vi "Init.vi"(8 "error in (no error)":errorcluster, 10 "model_v1_parameters":T1, 11 "OUR_Monitor in":refnum<class "OUR_Monitor.lvclass">) -> (0 "error out":errorcluster, 3 "OUR_Monitor out":refnum<class "OUR_Monitor.lvclass">)   [LabVIEW 2021, in "MBPOnOff_Controller.lvlib" / "OUR_Monitor.lvclass"]
uses:
  OUR_Monitor.lvclass
  Model_Predictor/typedefs/Model_v1_parameters.ctl
  OUR_Monitor.lvclass/OUR_Monitor.ctl
  Model_Predictor/Model_Predictor.lvclass
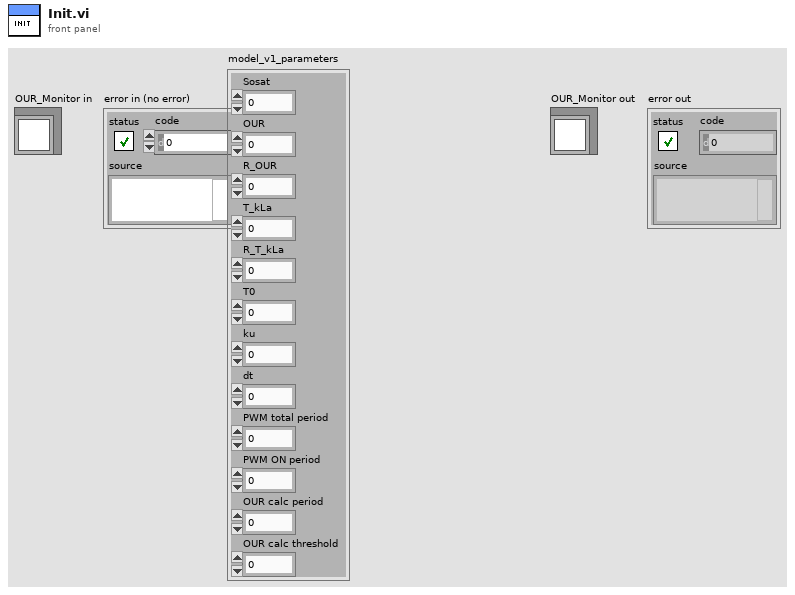
[diagram p1: front panel]
types:
  T1 = typedef "MBPOnOff_Controller.lvlib/Model_Predictor.lvclass/Model_v1_parameters.ctl" = cluster{"Sosat":dbl, "OUR":dbl, "R_OUR":dbl, "T_kLa":dbl, "R_T_kLa":dbl, "T0":dbl, "ku":dbl, "dt":dbl, "PWM total period":dbl, "PWM ON period":dbl, "OUR calc period":dbl, "OUR calc threshold":dbl}
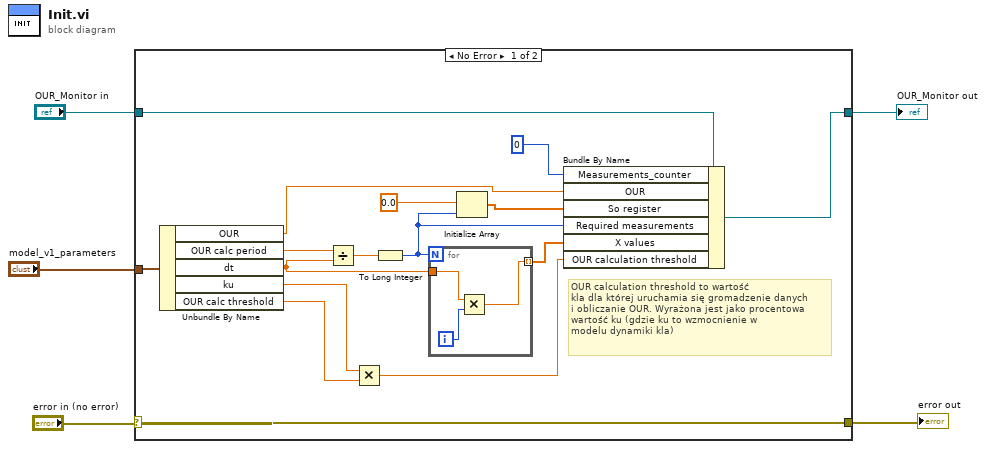
[diagram p0: block diagram]
diagram:
  n1 = case shown="No Error" "error in (no error)" {
    selector: "error in (no error)" -> [w21 w26]
    tunnel: [w21 w26] -> w4
    tunnel: [w17 w25] -> w3
    tunnel: "OUR_Monitor in" -> [w20 w25]
    tunnel: "model_v1_parameters" -> [w11 _]
    frame No Error {
      # "OUR calculation threshold to wartość\nkla dla której uruchamia się gromadzenie danych\ni obliczanie OUR. Wyrażona jest jako procentowa \nwartość ku (gdzie ku to wzmocnienie w\nmodelu dynamiki kla)"
      n2 = Unbundle By Name(w11) -> ("OUR"=w10:dbl, "OUR calc period"=w9:dbl, "dt"=w6:dbl, "ku"=w8:dbl, "OUR calc threshold"=w7:dbl)
      n3 = Divide(x=w9, y=w6) -> (x/y=w18:dbl)
      n4 = Multiply(x=w8, y=w7) -> (x*y=w12:dbl)
      n5 = To Long Integer(number=w18) -> (32bit integer=w14:i32)
      n6 = for {
        N: w14 -> [_]
        tunnel: [w23] -> w13 mode=indexing
        tunnel: w6 -> [w22]
        i -> [w24]
        n7 = Multiply(x=w22, y=w24) -> (x*y=w23:dbl)
      }
      n8 = Initialize Array(0.0 ("element"), w14) -> (w15:dbl[])
      n9 = Bundle By Name(cluster=w20, "Measurements_counter"=0, "OUR"=w10, "So register"=w15, "Required measurements"=w14, "X values"=w13, "OUR calculation threshold"=w12) -> (w17:refnum<class "OUR_Monitor.lvclass">)
    }
    frame Error {
    }
  }
  "OUR_Monitor out" <- w3
  "error out" <- w4
